vi "integration.vi"(9 "rt":dbl, 10 "dist":dbl, 11 "pos(i-1)":dbl[](array[numeric])) -> (3 "pos(i)":dbl[](array[numeric]))   [LabVIEW 2012]
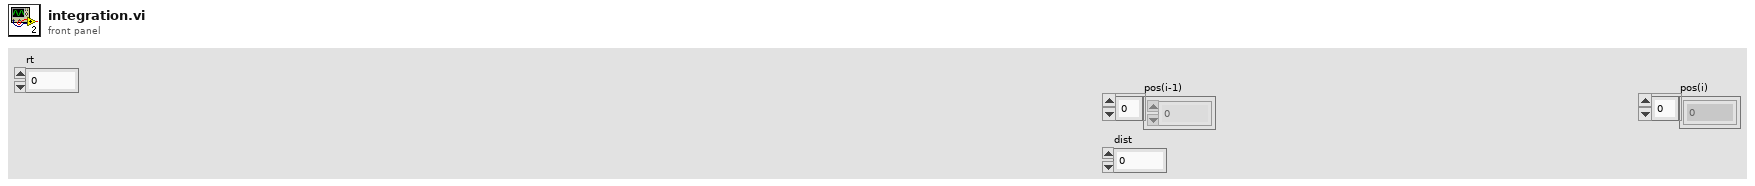
[diagram p1: front panel]
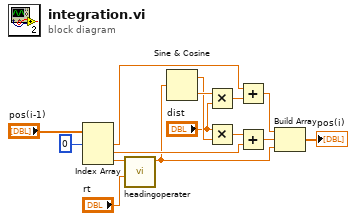
[diagram p0: block diagram]
diagram:
  n1 = Index Array(array="pos(i-1)", index #1=0 ("index")) -> (element #1=w13:dbl, element #2=w11:dbl, element #3=w8:dbl)  [unwired: 2 in]
  n2 = call "headingoperater.vi"("h1"="rt", "h2"=w8) -> ("h2+h1"=w7:dbl)  [unwired: 8 in, 1 out]
  n3 = Sine & Cosine(0:w7) -> (1:w5:dbl, 2:w6:dbl)
  n4 = Multiply(x=w6, y="dist") -> (x*y=w14:dbl)
  n5 = Multiply(x="dist", y=w5) -> (x*y=w12:dbl)
  n6 = Add(x=w13, y=w14) -> (x+y=w10:dbl)
  n7 = Add(x=w12, y=w11) -> (x+y=w9:dbl)
  n8 = Build Array(w10, w9, w7) -> (→"pos(i)":dbl[])
